vi "Acq Convert To Waveform.vi"(0 "session in":refnum<class "Digitizer Control.lvclass">, 1 "sample data":i16[](array[numeric]), 5 "error in (no error)":errorcluster, 8 "channel index":i32) -> (14 "session out":refnum<class "Digitizer Control.lvclass">, 15 "waveform (V)":waveform(dbl), 19 "error out":errorcluster)   [LabVIEW 2021, in "Digitizer Control.lvclass"]
doc: "Converts the IQ data array of I16s transferred by the FPGA Target to a waveform.\n\nInputs:\n\n<B>session in</B>: The device session.\n\n<B>channel index</B>: The index of the channel whose format the array passed on the <B>sample data</B> input is using.\n\n<B>sample data</B>: The sample data as an array of I16s. This VI assumes that the data in the array starts at sample boundary.\n\nOutputs:\n\n<B>session out</B>: The device session passed on the <B>session in</B> input.\n\n<B>waveform</B>: The waveform scaled to Volts."
uses:
  Digitizer Control.lvclass
  Digitizer Control.lvclass/Digitizer Control.ctl
  <vilib>/Utility/error.llb/Error Cluster From Error Code.vi
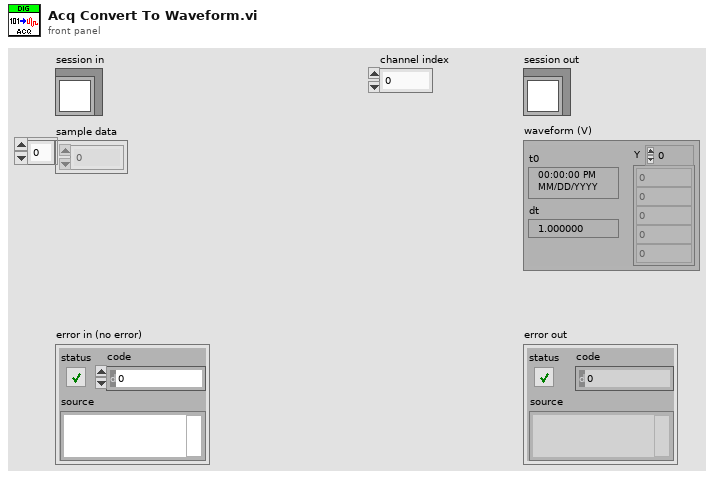
[diagram p1: front panel]
types:
  T1 = typedef "Digitizer Control.lvclass/Acq Session Data.ctl" = cluster{"ADC sampling rate":dbl, "SCTL rate":dbl, "DMA element size (bits)":i32, "sample size (bits)":i32[], "DMA/memory interface width (DMA elements)":i32, "transfer size (bits)":i32[], "stream instance":i32[], "trigger instance":u32, "group delay (s)":dbl, "data delay (s)":dbl, "target delay (s)":dbl, "trigger tracking enabled":bool, "channel configured":bool, "enabled channels":bool[], "transfer configured":bool, "dsp bypass":bool, "fractional decimator input rate":dbl, "fractional decimator output rate":dbl, "sample scale factor":dbl[], "memory size":u64[], "FIFO size":u64}
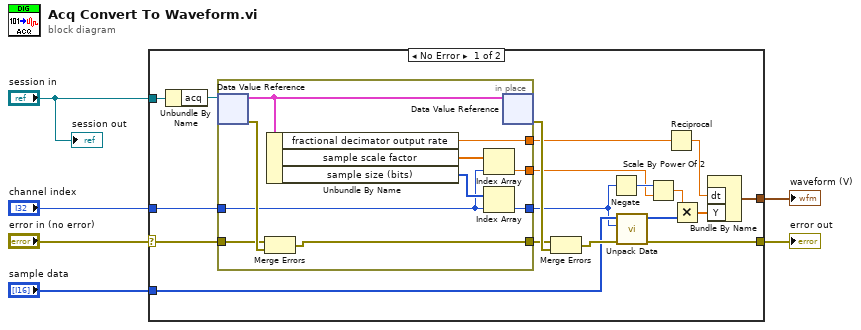
[diagram p0: block diagram]
diagram:
  n1 = case shown="No Error" "error in (no error)" {
    selector: "error in (no error)" -> [w21 w35]
    tunnel: [w14 w35] -> w3
    tunnel: [w23 _] -> w5
    tunnel: "session in" -> [w18 _]
    tunnel: "sample data" -> [w10 _]
    tunnel: "channel index" -> [w9 _]
    frame No Error {
      n2 = Unbundle By Name(w18) -> ("acq"=w17:refnum<data-value>)
      n3 = in-place {
        in-place-border: w21 -> [w33]
        in-place-border: [w31] -> w12
        in-place-border: [w26] -> w13
        in-place-border: [w29] -> w20
        in-place-border: [w27] -> w8
        in-place-border: w9 -> [w25]
        n4 = in-place-dvr #1(w17) -> (w32:T1, w34:errorcluster)
        n5 = Merge Errors(w33, w34) -> (w29:errorcluster)
        n6 = Unbundle By Name(w32) -> ("fractional decimator output rate"=w31:dbl, "sample scale factor"=w30:dbl[], "sample size (bits)"=w28:i32[])
        n7 = Index Array(array=w30, index=w25) -> (element=w26:dbl)
        n8 = Index Array(array=w28, index=w25) -> (element=w27:i32)
        n9 = in-place-dvr #1(w32) -> (w24:errorcluster)  [unwired: 1 out]
      }
      n10 = Merge Errors(w20, w24) -> (w11:errorcluster)
      n11 = Negate(x=w8) -> (-x=w16:i32)
      n12 = call "Unpack Data.vi"("error in (no error)"=w11, "packed data size (bits)"=w8, "packed data in"=w10) -> ("error out"=w14:errorcluster, "unpacked data out"=w7:i16[])  [unwired: 7 in]
      n13 = Scale By Power Of 2(n=w16, x=w13) -> (x*2^n=w15:dbl)
      n14 = Reciprocal(x=w12) -> (1/x=w19:dbl)
      n15 = Multiply(x=w15, y=w7) -> (x*y=w22:dbl[])
      n16 = Bundle By Name("dt"=w19, "Y"=w22) -> (w23:waveform(dbl))  [unwired: 1 in]
    }
    frame Error {
    }
  }
  "waveform (V)" <- w5
  "error out" <- w3
  "session out" <- "session in"
